vi "Get Property.vi"(7 "MsgSerializer":refnum<class "MsgSerializer.lvclass">, 10 "Property":variant) -> (2 "Properties":T1[](array[typedef]))   [LabVIEW 2013, in "JUnit for Azure Pipelines.lvclass"]
uses:
  JUnit for Azure Pipelines.lvclass
  <vilib>/addons/_JKI Toolkits/Caraya/classes/MsgSerializer/MsgSerializer.lvclass
  Test Case Property.ctl
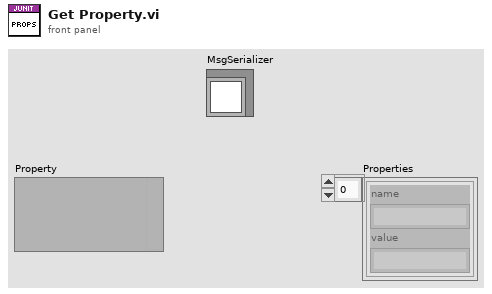
[diagram p1: front panel]
types:
  T1 = typedef "JUnit for Azure Pipelines.lvclass/Test Case Property.ctl" = cluster{"name":string, "value":string}
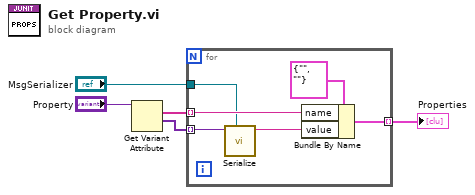
[diagram p0: block diagram]
diagram:
  n1 = Get Variant Attribute(Variant="Property") -> (names=w5:string[], values=w4:variant[])  [unwired: 3 in, 2 out]
  n2 = for {
    tunnel: w5 -> [w10] mode=indexing
    tunnel: w4 -> [w8] mode=indexing
    tunnel: [w9] -> w1 mode=indexing
    tunnel: "MsgSerializer" -> [w6]
    n3 = call-dynamic "Serialize.vi"("MsgSerializer"=w6, "Value"=w8) -> ("Serialized Message"=w7:string)  [unwired: 8 in, 1 out]
    n4 = Bundle By Name(cluster=T1 {"name"="", "value"=""} ("Property"), "name"=w10, "value"=w7) -> (w9:T1)
  }
  "Properties" <- w1
